vi "go postion.vi"(11 "get and go Position in":T1) -> (1 "XY(F)/XYZ(T)":bool, 2 "Array out":dbl[](array[numeric]), 3 "get and go Position out":T1)   [LabVIEW 2016]
panel:
  out "insert output array":dbl[](array[numeric])
  out "subarray":dbl[](array[numeric])
  out "appended array":i32[](array[numeric])
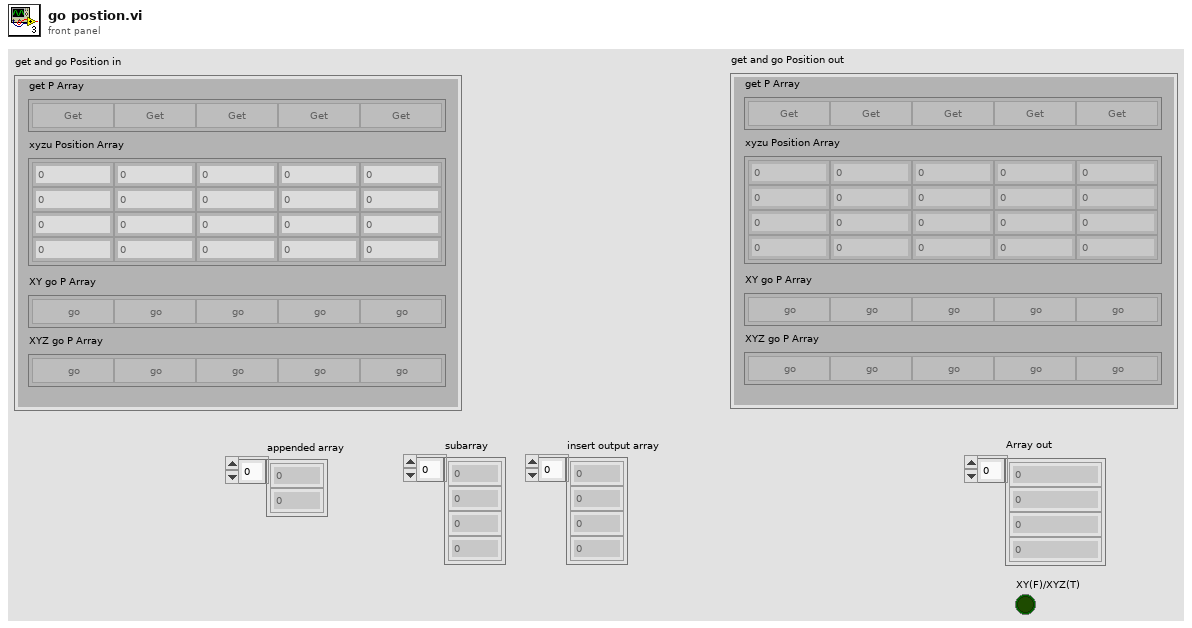
[diagram p1: front panel]
types:
  T1 = cluster{"get P Array":bool[], "XY go P Array":bool[], "xyzu Position Array":dbl[][], "XYZ go P Array":bool[]}
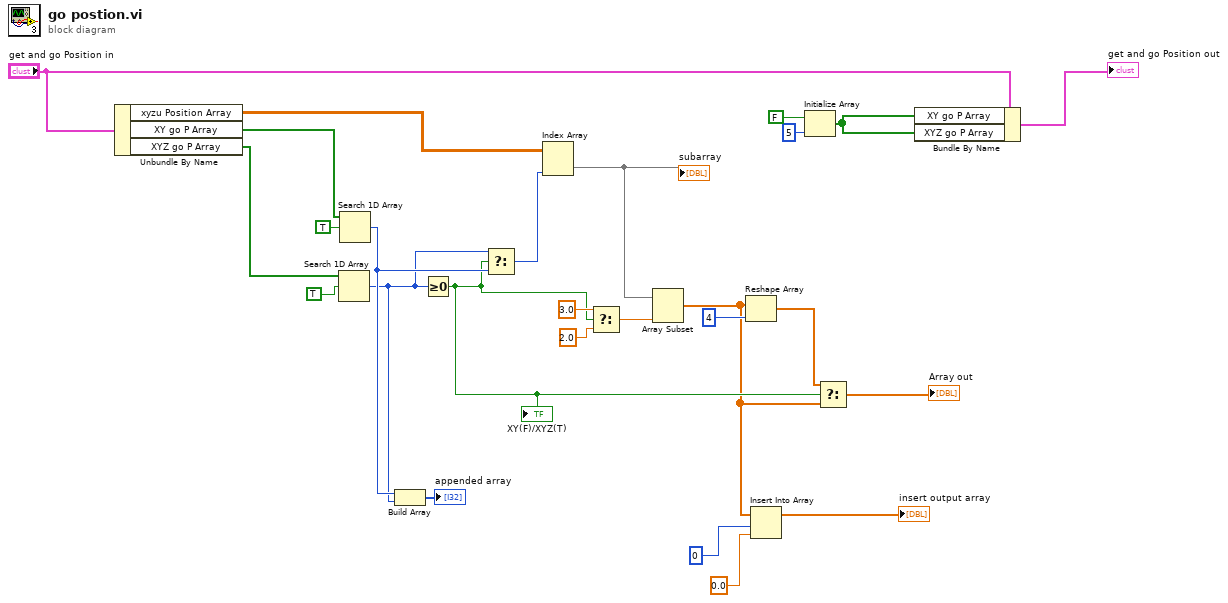
[diagram p0: block diagram]
diagram:
  n1 = Unbundle By Name("get and go Position in") -> ("xyzu Position Array"=w22:dbl[][], "XY go P Array"=w26:bool[], "XYZ go P Array"=w23:bool[])
  n2 = Search 1D Array(1D array=w23, element=TRUE) -> (index of element=w19:i32)  [unwired: 1 in]
  n3 = Search 1D Array(1D array=w26, element=TRUE) -> (index of element=w20:i32)  [unwired: 1 in]
  n4 = Build Array(w20, w19) -> (→"appended array":i32[])
  n5 = Greater Or Equal To 0?(x=w19) -> (x >= 0?=w9:bool)
  "XY(F)/XYZ(T)" <- w9
  n6 = Select(t=w19, s=w9, f=w20) -> (s? t:f=w18:i32)
  n7 = Index Array(array=w22, index (col)=w18) -> (element=w15:dbl[])  [unwired: 1 in]
  "subarray" <- w15
  n8 = Select(t=3.0, s=w9, f=2.0 ("t")) -> (s? t:f=w14:dbl)
  n9 = Array Subset "Array Subset"(array=w15, length=w14) -> (w8:dbl[])  [unwired: 1 in]
  n10 = Reshape Array "Reshape Array"(w8, 4 ("index")) -> (w7:dbl[])
  n11 = Insert Into Array "Insert Into Array"(array=w8, index=0, new element=0.0 ("new element/subarray")) -> (→"insert output array":dbl[])
  n12 = Initialize Array(FALSE, 5 ("dimension size")) -> (w1:bool[])
  n13 = Select(t=w7, s=w9, f=w8) -> (s? t:f=→"Array out":dbl[])
  n14 = Bundle By Name(cluster="get and go Position in", "XY go P Array"=w1, "XYZ go P Array"=w1) -> (→"get and go Position out":T1)
